vi "measurements to graph.vi"(9 "index":i32, 10 "measurements":T1(array[cluster])) -> (2 "graph values":cluster{dbl, "pid reading":dbl}[](array[cluster]))   [LabVIEW 2013]
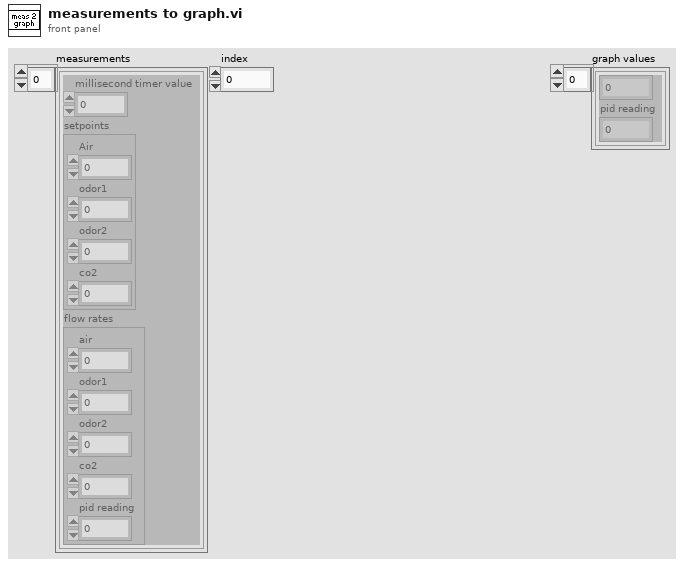
[diagram p1: front panel]
types:
  T1 = cluster{"millisecond timer value":u32, "setpoints ":cluster{"Air ":dbl, "odor1":dbl, "odor2":dbl, "co2":dbl}, "flow rates":cluster{"air":dbl, "odor1":dbl, "odor2":dbl, "co2":dbl, "pid reading":dbl}}[]
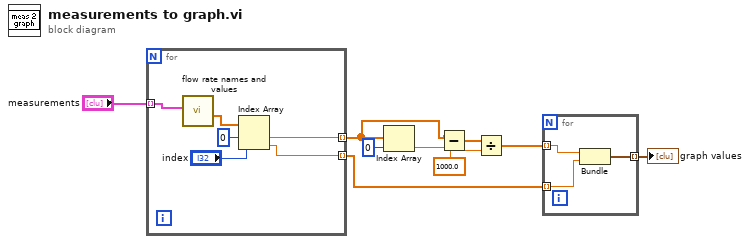
[diagram p0: block diagram]
diagram:
  n1 = for {
    tunnel: "measurements" -> [w15] mode=indexing
    tunnel: [w11] -> w6 mode=indexing
    tunnel: [w10] -> w3 mode=indexing
    n2 = call "flow rate names and values.vi"("measurements"=w15) -> ("values"=w14:dbl[])  [unwired: 9 in, 1 out]
    n3 = Index Array(array=w14, index #1=0 ("index"), index #2="index") -> (element #1=w11:dbl, element #2=w10:dbl)
  }
  n4 = Index Array(array=w6, index=0) -> (element=w7:dbl)
  n5 = Subtract(x=w6, y=w7) -> (x-y=w5:dbl[])
  n6 = Divide(x=w5, y=1000.0) -> (x/y=w2:dbl[])
  n7 = for {
    tunnel: w3 -> [w17] mode=indexing
    tunnel: w2 -> [w18] mode=indexing
    tunnel: [w16] -> w1 mode=indexing
    n8 = Bundle(w18, "pid reading"=w17) -> (w16:cluster{dbl, "pid reading":dbl})  [unwired: 1 in]
  }
  "graph values" <- w1
